vi "Library Name Cut.vi"(9 "Cut? (T)":bool=TRUE, 11 "Name in":string) -> (3 "Name out":string)   [LabVIEW 2023, in "VIDoc Printer - Confluence.lvlib" / "VIDoc Printer - Confluence.lvclass"]
uses:
  VIDoc Printer - Confluence.lvclass
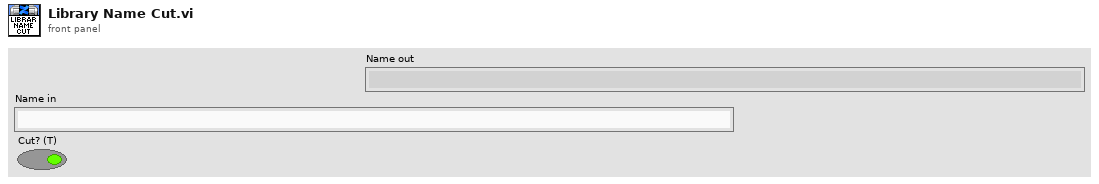
[diagram p1: front panel]
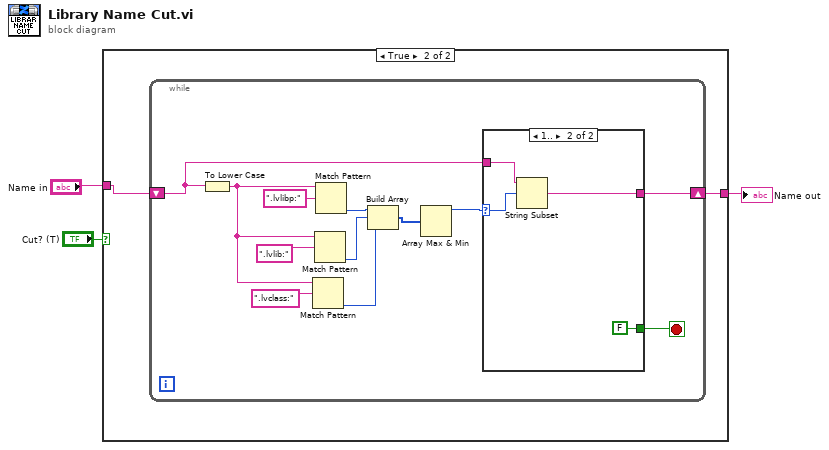
[diagram p0: block diagram]
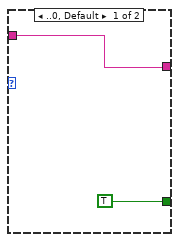
[diagram p3: hidden frame]
diagram:
  n1 = case shown="True" "Cut? (T)" {
    tunnel: [w4 w6] -> w3
    tunnel: "Name in" -> [w4 w5]
    frame False {
    }
    frame True {
      n2 = while {
        shift-right: [w10] -> w6
        shift-left: w5 -> [w9]
        stop <- w8 stop-if-true
        n3 = To Lower Case(string=w9) -> (all lower case string=w18:string)
        n4 = Match Pattern(string=w18, regular expression=".lvclass:") -> (offset past match=w12:i32)  [unwired: 1 in, 3 out]
        n5 = Match Pattern(string=w18, regular expression=".lvlib:") -> (offset past match=w13:i32)  [unwired: 1 in, 3 out]
        n6 = Match Pattern(string=w18, regular expression=".lvlibp:") -> (offset past match=w14:i32)  [unwired: 1 in, 3 out]
        n7 = Build Array(w14, w13, w12) -> (w11:i32[])
        n8 = Array Max & Min(array=w11) -> (max value=w7:i32)  [unwired: 3 out]
        n9 = case shown="1.." w7 {
          selector: w7 -> [_ w23]
          tunnel: w9 -> [w20 w24]
          tunnel: [w20 w22] -> w10
          tunnel: [TRUE FALSE] -> w8
          frame ..0, Default {
          }
          frame 1.. {
            n10 = String Subset(string=w24, offset (0)=w23) -> (substring=w22:string)  [unwired: 1 in]
          }
        }
      }
    }
  }
  "Name out" <- w3
